vi "Write Meta Data.vi"(8 "error in (no error)":errorcluster, 10 "report in":refnum<class "NI_report.lvclass">, 11 "Hardware Resources in":T1={"Test Setting"={"Test_Num"=0, "Test_ID"=0, "Proc_ID"=0, "Max Force"=0.0, "User"="", "SN"="", "Date"=""}, "Measurements"=[[""]], "LOG REF"=refnum, "Report Template"=path "", "Save Report path"=path "", "Data File Path"=path "", "Popup Dialog"=FALSE}) -> (0 "error out":errorcluster, 2 "report out":refnum<class "NI_report.lvclass">, 3 "Hardware Resources out":T1)   [LabVIEW 2020, in "Report.lvlib"]
doc: "Perform the acquisition. Replace the contents of this diagram with calls to acquisition hardware."
uses:
  Report.lvlib
  REP Configuration.ctl
  Test Setting.ctl
  <vilib>/Utility/NIReport.llb/NI_report.lvclass
  <vilib>/Utility/NIReport.llb/Append Report Text (str wrap).vi
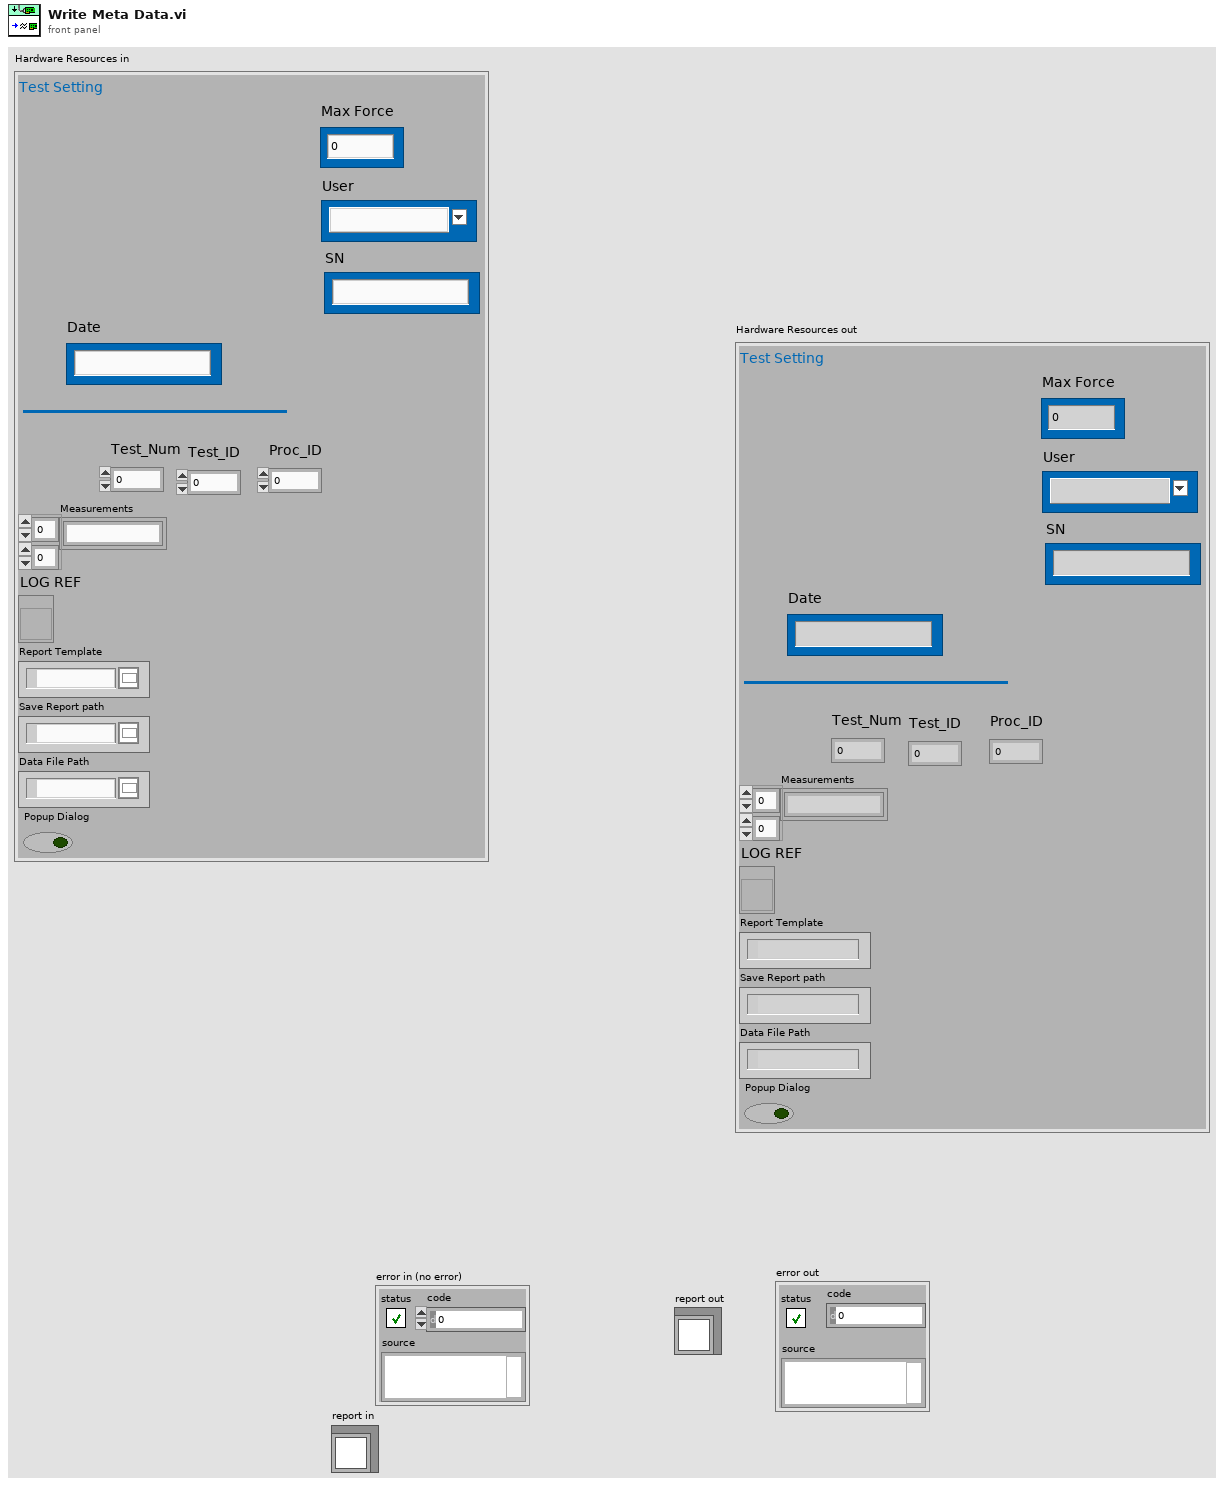
[diagram p1: front panel]
types:
  T1 = typedef "Report.lvlib/REP Configuration.ctl" = cluster{"Test Setting":T2, "Measurements":string[][], "LOG REF":refnum<vi>, "Report Template":path, "Save Report path":path, "Data File Path":path, "Popup Dialog":bool}
  T2 = typedef "Report.lvlib/Test Setting.ctl" = cluster{"Test_Num":i32, "Test_ID":i32, "Proc_ID":i32, "Max Force":dbl, "User":string, "SN":string, "Date":string}
  T3 = cluster{"position (excel)":cluster{"row":i32, "column":i32}, "name (excel)":string, "bookmark (word)":string}
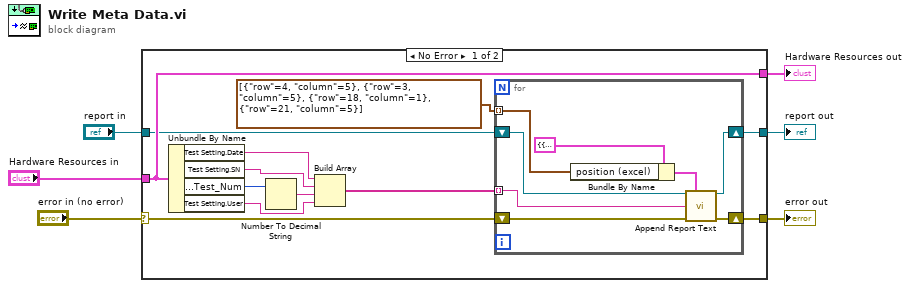
[diagram p0: block diagram]
diagram:
  n1 = case shown="No Error" "error in (no error)" {
    selector: "error in (no error)" -> [w13 w28]
    tunnel: [w15 w28] -> w5
    tunnel: "Hardware Resources in" -> [w18 w29]
    tunnel: [w18 w29] -> w3
    tunnel: "report in" -> [w17 w27]
    tunnel: [w16 w27] -> w1
    frame No Error {
      n2 = Unbundle By Name(w18) -> ("Test Setting.Date"=w7:string, "Test Setting.SN"=w11:string, "Test Setting.Test_Num"=w10:i32, "Test Setting.User"=w8:string)
      n3 = Number To Decimal String(number=w10) -> (decimal integer string=w9:string)  [unwired: 1 in]
      n4 = Build Array(w7, w11, w9, w8) -> (w14:string[])
      n5 = for {
        shift-right: [w24] -> w16
        shift-left: w17 -> [w26]
        shift-right: [w23] -> w15
        shift-left: w13 -> [w25]
        tunnel: w14 -> [w21] mode=indexing
        tunnel: cluster{"row":i32, "column":i32}[] [{"row"=4, "column"=5}, {"row"=3, "column"=5}, {"row"=18, "column"=1}, {"row"=21, "column"=5}] -> [w19] mode=indexing
        n6 = Bundle By Name(cluster=T3 {"position (excel)"={"row"=0, "column"=0}, "name (excel)"="", "bookmark (word)"=""} ("MS Office parameters"), "position (excel)"=w19) -> (w22:T3)
        n7 = call-poly <vilib>:"Append Report Text.vi"("report in"=w26, "MS Office parameters"=w22, "text"=w21, "error in (no error)"=w25) -> ("report out"=w24:refnum<class "NI_report.lvclass">, "error out"=w23:errorcluster)  [unwired: 8 in, 2 out]
      }
    }
    frame Error {
    }
  }
  "Hardware Resources out" <- w3
  "error out" <- w5
  "report out" <- w1
